vi "Set Level.vi"(8 "error in (no error)":errorcluster, 10 "Setpoint":dbl min=0.0 max=16.0 step=0.5 format="%04.1f", 11 "SS P100 Settings In":T1) -> (0 "error out":errorcluster, 1 "Connection Error":bool, 3 "SS P100 Settings Out":T1)   [LabVIEW 2018, in "Sonic Systems P100.lvlib"]
uses:
  Sonic Systems P100.lvlib
  Sonic Systems P100 Settings.ctl
  support/Support Library.lvlib
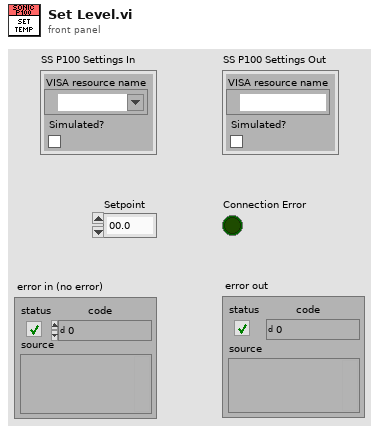
[diagram p1: front panel]
types:
  T1 = typedef "Sonic Systems P100.lvlib/Sonic Systems P100 Settings.ctl" = cluster{"VISA resource name":refnum<visa-resource-name>, "Simulated?":bool}
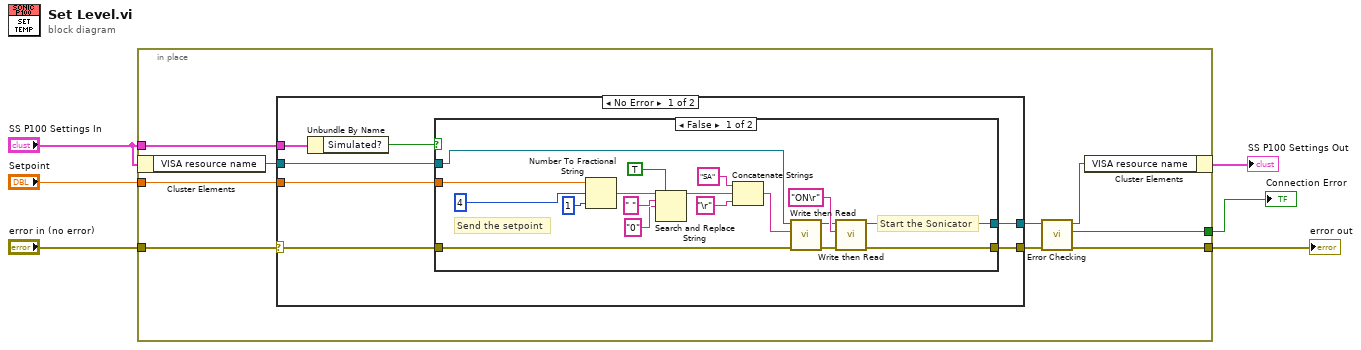
[diagram p0: block diagram]
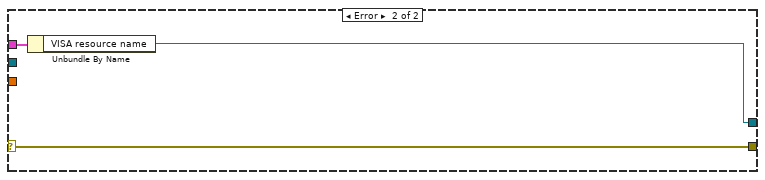
[diagram p3: hidden frame]
diagram:
  n1 = in-place {
    in-place-border: "error in (no error)" -> [w15]
    in-place-border: "SS P100 Settings In" -> [w12]
    in-place-border: "Setpoint" -> [w11]
    in-place-border: [w10] -> w4
    in-place-border: [w9] -> w3
    n2 = in-place-cluster #1("SS P100 Settings In") -> ("VISA resource name"=w8:refnum<visa-resource-name>)
    n3 = case shown="No Error" w15 {
      selector: w15 -> [w22 w45]
      tunnel: w12 -> [w18 w44]
      tunnel: [w21 w45] -> w13
      tunnel: [w20 w43] -> w14
      tunnel: w11 -> [w17 _]
      tunnel: w8 -> [w16 _]
      frame No Error {
        n4 = Unbundle By Name(w18) -> ("Simulated?"=w19:bool)
        n5 = case shown="False" w19 {
          tunnel: w22 -> [w34 w42]
          tunnel: [w30 w42] -> w21
          tunnel: [w29 w41] -> w20
          tunnel: w16 -> [w35 w41]
          tunnel: w17 -> [w38 _]
          frame False {
            # "Start the Sonicator"
            # "Send the setpoint"
            n6 = Number To Fractional String(number=w38, width (-)=i16 4, precision (6)=i16 1) -> (F-format string=w24:string)  [unwired: 1 in]
            n7 = Search and Replace String(replace all?=TRUE ("replace all? (F)"), input string=w24, search string=" ", replace string="0" ("replace string (\"\")")) -> (result string=w23:string)  [unwired: 4 in, 3 out]
            n8 = Concatenate Strings("SA" ("string"), w23, "\r" ("string")) -> (w28:string)
            n9 = call "Write then Read.vi"("error in"=w34, "write buffer"=w28, "VISA resource name in"=w35) -> ("error out"=w31:errorcluster, "VISA resource name out"=w32:refnum<visa-resource-name>)  [unwired: 6 in, 1 out]
            n10 = call "Write then Read.vi"("error in"=w31, "write buffer"="ON\r", "VISA resource name in"=w32) -> ("error out"=w30:errorcluster, "VISA resource name out"=w29:refnum<visa-resource-name>)  [unwired: 6 in, 1 out]
          }
          frame True {
          }
        }
      }
      frame Error {
        n11 = Unbundle By Name(w44) -> ("VISA resource name"=w43:refnum<visa-resource-name>)
      }
    }
    n12 = call "Error Checking.vi"("error in (no error)"=w13, "VISA resource name"=w14) -> ("error out"=w9:errorcluster, "Connection Error"=w10:bool, "VISA resource name"=w7:refnum<visa-resource-name>)  [unwired: 7 in]
    n13 = in-place-cluster #1("VISA resource name"=w7) -> (→"SS P100 Settings Out":T1)
  }
  "error out" <- w3
  "Connection Error" <- w4
